vi "ast_build.vi"(7 "query_type":T1, 8 "error in (no error)":errorcluster, 11 "term":string) -> (0 "error out":errorcluster, 3 "query":string)   [LabVIEW 2017, in "rethinkdb.lvlib"]
uses:
  rethinkdb.lvlib
  ql2_query.ctl
  ql2_query_to_id.vi
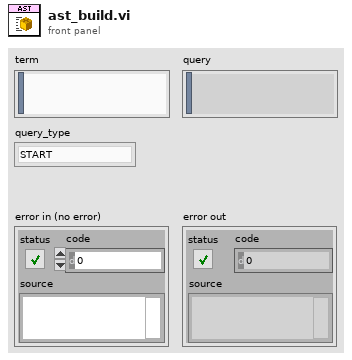
[diagram p1: front panel]
types:
  T1 = typedef "rethinkdb.lvlib/ql2_query.ctl" = enum8{"START", "CONTINUE", "STOP", "NOREPLY_WAIT", "SERVER_INFO", "invalid"}
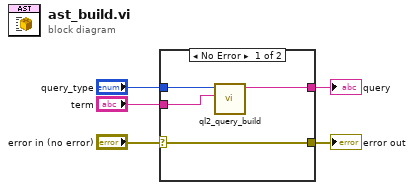
[diagram p0: block diagram]
diagram:
  n1 = case shown="No Error" "error in (no error)" {
    selector: "error in (no error)" -> [w9 w10]
    tunnel: [w6 _] -> w5
    tunnel: [w9 w10] -> w4
    tunnel: "term" -> [w8 _]
    tunnel: "query_type" -> [w7 _]
    frame No Error {
      n2 = call "ql2_query_build.vi"("term"=w8, "query_type"=w7) -> ("query"=w6:string)  [unwired: 9 in]
    }
    frame Error {
    }
  }
  "query" <- w5
  "error out" <- w4
